vi "get runtime class name.vi"(8 "error in":errorcluster, 11 "module configuration in":refnum<class "TBM module configuration.lvclass">) -> (0 "error out":errorcluster, 2 "class name":string, 3 "module configuration out":refnum<class "TBM module configuration.lvclass">)   [LabVIEW 2013, in "TBM module configuration.lvclass"]
doc: "Provides an interface for determining the module runtime class associated with this module configuration. This class name can then be used to dynamically load or locate the runtime class for initialization purposes."
uses:
  TBM module configuration.lvclass
  <vilib>/NI/Configuration Framework/NISE_CEF_TreeControl.lvlib
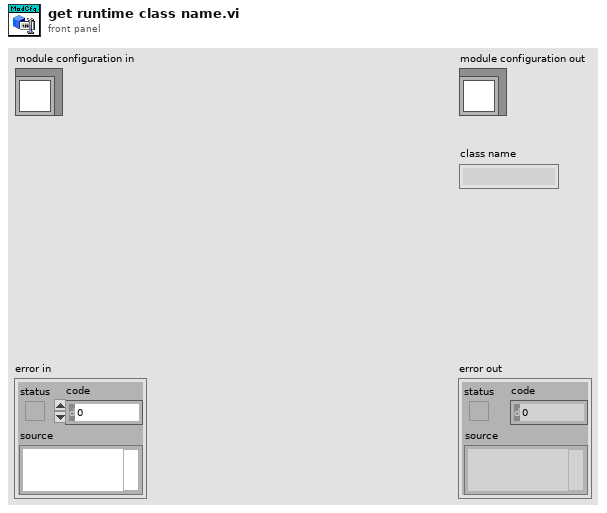
[diagram p1: front panel]
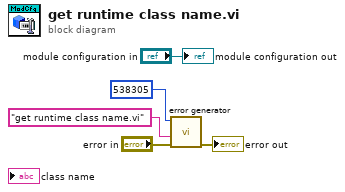
[diagram p0: block diagram]
diagram:
  n1 = call <vilib>:"error generator.vi"("error in"="error in", "source"="get runtime class name.vi", "error code (0)"=538305) -> ("error out"=→"error out":errorcluster)  [unwired: 6 in]
  "module configuration out" <- "module configuration in"
